vi "plc debug.vi"() -> ()   [LabVIEW 2020]
uses:
  Type Defs/Modbus Mode.ctl
  Type Defs/PLC Coils.ctl
  Type Defs/PLC Registers.ctl
  Type Defs/HMI Coils.ctl
  Type Defs/HMI Registers.ctl
panel:
  in  "Speed CMD":u16
  out "Speed":u16
  out "Error OUT":errorcluster
  out "Registers OUT":u16[](array[numeric])
  out "Coils OUT":bool[](array[boolean])
  out "Overload":bool
  out "Running":bool
  in  "Wet Silo Drag":bool
  out "x-y":u32
  in  "stop":bool
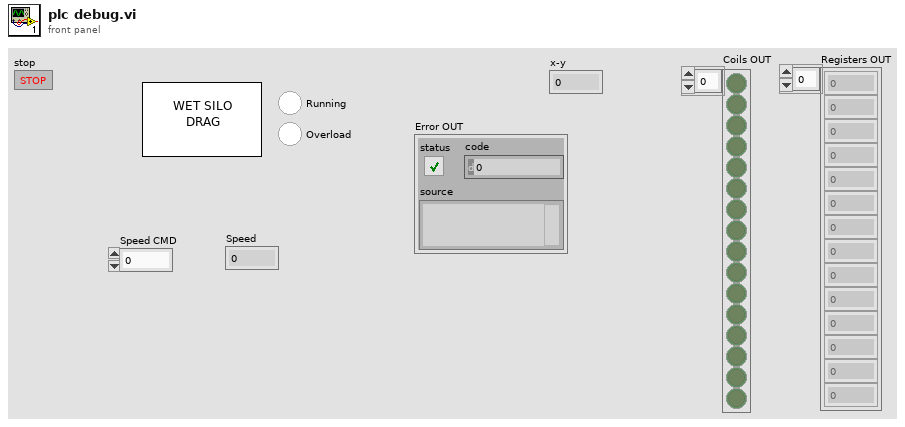
[diagram p1: front panel]
types:
  T1 = typedef "Modbus Mode.ctl" = enum16{"Init", "Read", "Write Coil", "Write Reg", "Close"}
  T2 = typedef "HMI Coils.ctl" = enum16{"C100_HMI_WS_Drag_PB", "C101_HMI_WB_Drag_PB", "C102_HMI_WS_Fan_PB", "C103_HMI_WB_Fan_PB", "C104_HMI_Dryr_Drag_PB", "C105_HMI_Dryr_Fan_PB", "C106_HMI_DB_Fan_PB", "C107_HMI_DB_Drag_PB", "C108_HMI_DB_Top_Feed_PB", "C109_HMI_U-Trough_PB", "C110_HMI_Leg_PB", "C111", "C112", "C113", "C114", "C115", "C116", "C117", "C118", "C119", "C220_HMI_VFD_+100_PB", "C221_HMI_VFD_+10_PB", "C222_HMI_VFD_-10_PB", "C223_HMI_VFD_-100_PB"}
  T3 = typedef "HMI Registers.ctl" = enum16{"V100_HMI_DB_Fan_CMD", "V101_HMI_DB_Drag_CMD", "V102_HMI_DB_TF_CMD", "V103_HMI_U-Trough_CMD", "V104_HMI_Leg_CMD", "V105_HMI_VFD_Select"}
  T4 = typedef "PLC Registers.ctl" = enum16{"V200_PLC_DB_Fan_Spd", "V201_PLC_DB_Drag_Spd", "V202_PLC_DB_Top_Fd_Spd", "V203_PLC_U-Trough_Spd", "V204_PLC_Leg_Spd", "V205", "V206", "V207", "V208", "V209", "V210", "V211_DB_Level", "V212_WB_Level", "V213_WS_Level"}
  T5 = typedef "PLC Coils.ctl" = enum16{"C200_PLC_Estop_Main", "C201_PLC_Estop_GSI", "C202_PLC_Estop_Dryer", "C203", "C204", "C205", "C206", "C207", "C208", "C209", "C210", "C211", "C212", "C213", "C214", "C215", "C216", "C217", "C218", "C219", "C220_PLC_WS_Drag_ON", "C221_PLC_WB_Drag_ON", "C222_PLC_WS_Fan_ON", "C223_PLC_WB_Fan_ON", "C224_PLC_Dryr_Drag_ON", "C225_PLC_Dryr_Fan_ON", "C226", "C227", "C228", "C229", "C230", "C231", "C232", "C233", "C234", "C235", "C236", "C237", "C238", "C239", "C240_PLC_WS_Drag_OL", "C241_PLC_WB_Drag_OL", "C242_PLC_WS_Fan_OL", "C243_PLC_WB_Fan_OL", "C244_PLC_Dryr_Drag_OL", "C245_PLC_Dryr_Fan_OL", "C246", "C247", "C248", "C249", "C250", "C251", "C252", "C253", "C254", "C255", "C256", "C257", "C258", "C259", "C260_PLC_Dryer_Full", "C261_PLC_Dryer_HI_Alm", "C262_PLC_DB_Full", "C263_PLC_DB_HI_Alm", "C264_PLC_Dryer_Chute", "C265_PLC_Dryer_Feed"}
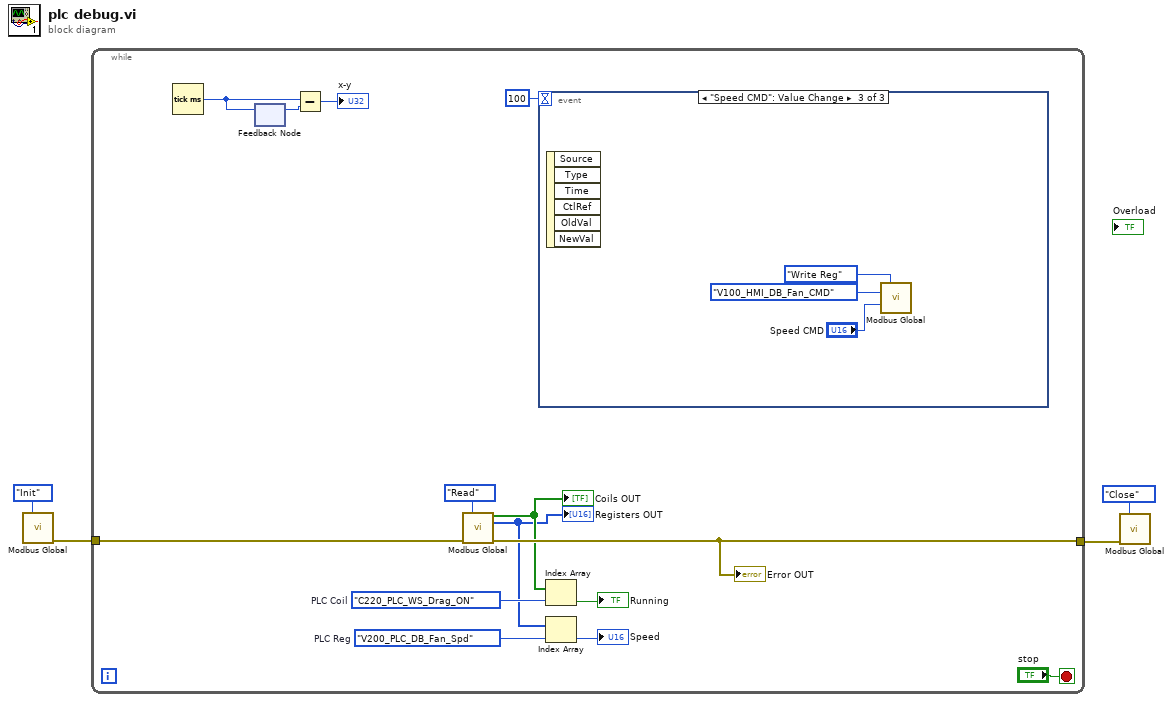
[diagram p0: block diagram]
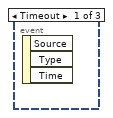
[diagram p2: hidden frame]
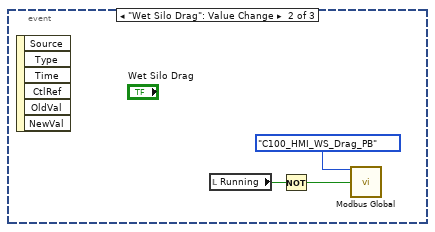
[diagram p3: hidden frame]
diagram:
  n1 = call "Modbus Global.vi"("Modbus Mode (Write Coil)"=Modbus_Mode."Init" ("Modbus Mode")) -> ("Error OUT"=w3:errorcluster)  [unwired: 12 in, 2 out]
  n2 = while {
    tunnel: w3 -> [w12]
    tunnel: [w11] -> w1
    stop <- "stop" stop-if-true
    w6 = PLC_Registers."V200_PLC_DB_Fan_Spd"  # PLC Reg
    w9 = PLC_Coils."C220_PLC_WS_Drag_ON"  # PLC Coil
    n3 = Tick Count (ms)() -> (millisecond timer value=w17:u32)
    n4 = feedback-in #1(w17) -> ()
    n5 = feedback #1() -> (w16:u32)  [unwired: 1 in]
    n6 = Subtract(x=w17, y=w16) -> (x-y=→"x-y":u32)
    n7 = call "Modbus Global.vi"("Modbus Mode (Write Coil)"=Modbus_Mode."Read" ("Modbus Mode"), "Error IN"=w12) -> ("Coils OUT"=w10:bool[], "Registers OUT"=w7:u16[], "Error OUT"=w11:errorcluster)  [unwired: 11 in]
    "Coils OUT" <- w10
    "Registers OUT" <- w7
    "Error OUT" <- w11
    n8 = event shown="[2] \"Speed CMD\": Value Change" {
      selector: _ -> [_ _ _]
      dyn-events: _ -> [_ _ _]
      timeout: 100 -> [_ _ _]
      event Timeout {
        n9 = event-data() -> ()  [unwired: 1 in, 3 out]
      }
      event "Wet Silo Drag": Value Change {
        n10 = event-data() -> ()  [unwired: 1 in, 6 out]
        n11 = local read "Running"() -> (w21:bool)
        n12 = Not(x=w21) -> (.not. x?=w19:bool)
        n13 = call "Modbus Global.vi"("HMI Coil"=HMI_Coils."C100_HMI_WS_Drag_PB", "Coil IN"=w19) -> ()  [unwired: 11 in, 3 out]
      }
      event "Speed CMD": Value Change {
        n14 = event-data() -> ()  [unwired: 1 in, 6 out]
        n15 = call "Modbus Global.vi"("Modbus Mode (Write Coil)"=Modbus_Mode."Write Reg", "HMI Reg"=HMI_Registers."V100_HMI_DB_Fan_CMD", "Reg Data IN"="Speed CMD") -> ()  [unwired: 10 in, 3 out]
      }
    }
    n16 = Index Array(array=w10, index=w9) -> (element=→"Running":bool)
    n17 = Index Array(array=w7, index=w6) -> (element=→"Speed":u16)
  }
  n18 = call "Modbus Global.vi"("Modbus Mode (Write Coil)"=Modbus_Mode."Close" ("Modbus Mode"), "Error IN"=w1) -> ()  [unwired: 11 in, 3 out]
